vi "2D Array Mean.vi"(11 "Image Pixels (U8)":u8[][](array[numeric])) -> (2 "mean":dbl)   [LabVIEW 2015]
uses:
  <vilib>/Analysis/baseanly.llb/Mean (DBL).vi
  <vilib>/Analysis/NI_AALBase.lvlib
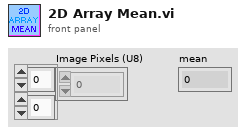
[diagram p1: front panel]
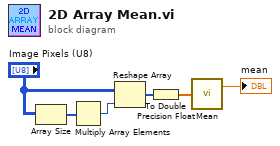
[diagram p0: block diagram]
diagram:
  n1 = Array Size(array="Image Pixels (U8)") -> (size(s)=w1:i32[])
  n2 = Multiply Array Elements(1:w1) -> (0:w2:i32)
  n3 = Reshape Array("Image Pixels (U8)", w2) -> (w4:u8[])
  n4 = To Double Precision Float(number=w4) -> (double precision float=w5:dbl[])
  n5 = call-poly <vilib>:"Mean.vi"("X"=w5) -> ("mean"=→"mean":dbl)  [unwired: 1 out]
